vi "create_material_experiment_lists.vi"(6 "Delimited Input String":string) -> (1 "Batch List by Material":string[](array[string]), 2 "Material Name List":string[](array[string]), 3 "Experiment Group Names List":string[](array[string]), 4 "Exerimement List by Group":string[](array[string]))   [LabVIEW 2015]
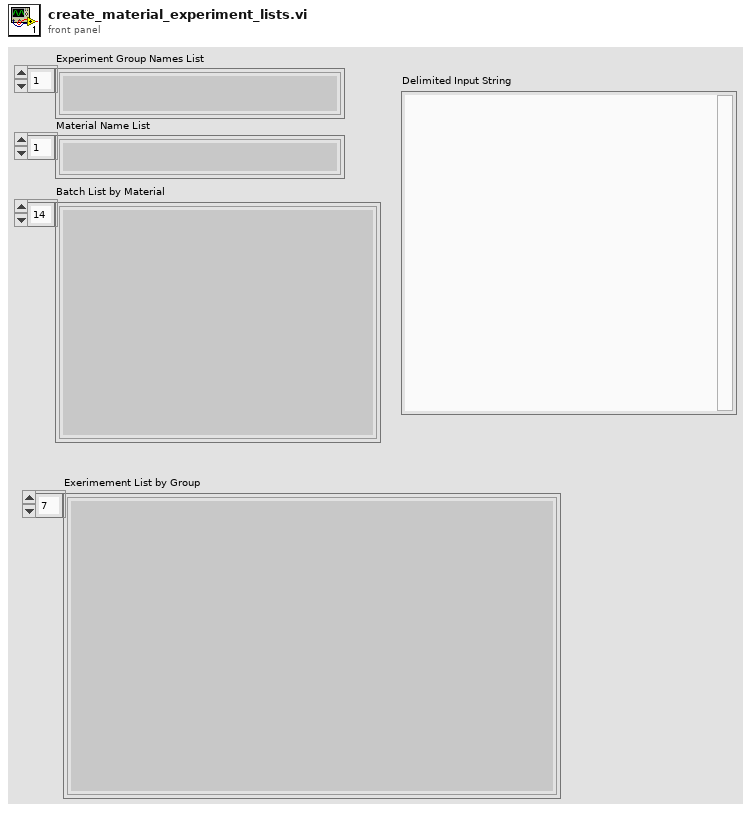
[diagram p1: front panel]
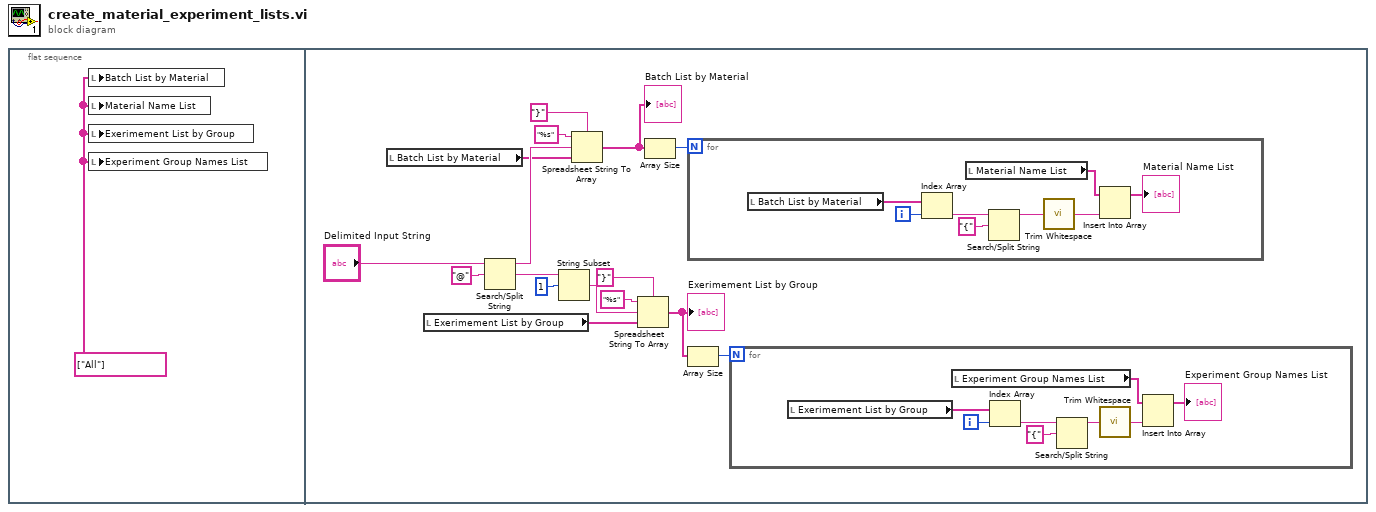
[diagram p0: block diagram]
diagram:
  n1 = flat-sequence {
    frame #0 {
      w1 = string[] ["All"]
      n2 = local write "Batch List by Material"(w1) -> ()
      n3 = local write "Material Name List"(w1) -> ()
      n4 = local write "Exerimement List by Group"(w1) -> ()
      n5 = local write "Experiment Group Names List"(w1) -> ()
    }
    frame #1 {
      n6 = local read "Batch List by Material"() -> (w10:string[])
      n7 = local read "Exerimement List by Group"() -> (w6:string[])
      n8 = Search/Split String(string="Delimited Input String", search string/char (-)="@") -> (substring before match=w13:string, match + rest of string=w14:string)  [unwired: 1 in, 1 out]
      n9 = String Subset(string=w14, offset (0)=1) -> (substring=w7:string)  [unwired: 1 in]
      n10 = Spreadsheet String To Array(delimiter (Tab)="}", format string="%s", spreadsheet string=w13, array type (2D Dbl)=w10) -> (array=w3:string[])
      "Batch List by Material" <- w3
      n11 = Spreadsheet String To Array(delimiter (Tab)="}", format string="%s", spreadsheet string=w7, array type (2D Dbl)=w6) -> (array=w2:string[])
      "Exerimement List by Group" <- w2
      n12 = Array Size(array=w3) -> (size(s)=w4:i32)
      n13 = for {
        N: w4 -> [_]
        i -> [w29]
        n14 = local read "Batch List by Material"() -> (w30:string[])
        n15 = Index Array(array=w30, index=w29) -> (element=w28:string)
        n16 = local read "Material Name List"() -> (w33:string[])
        n17 = Search/Split String(string=w28, search string/char (-)="{") -> (substring before match=w27:string)  [unwired: 1 in, 2 out]
        n18 = call <vilib>:"Trim Whitespace.vi"("string"=w27) -> ("trimmed string"=w26:string)  [unwired: 1 in]
        n19 = Insert Into Array(array=w33, new element=w26) -> (→"Material Name List":string[])  [unwired: 1 in]
      }
      n20 = Array Size(array=w2) -> (size(s)=w5:i32)
      n21 = for {
        N: w5 -> [_]
        i -> [w22]
        n22 = local read "Exerimement List by Group"() -> (w25:string[])
        n23 = local read "Experiment Group Names List"() -> (w21:string[])
        n24 = Index Array(array=w25, index=w22) -> (element=w23:string)
        n25 = Search/Split String(string=w23, search string/char (-)="{") -> (substring before match=w19:string)  [unwired: 1 in, 2 out]
        n26 = call <vilib>:"Trim Whitespace.vi"("string"=w19) -> ("trimmed string"=w18:string)  [unwired: 1 in]
        n27 = Insert Into Array(array=w21, new element=w18) -> (→"Experiment Group Names List":string[])  [unwired: 1 in]
      }
    }
  }
